vi "click on control.vi"(8 "error in (no error)":errorcluster, 10 "Reference to Button":refnum<vi>, 11 "VI Reference":refnum<vi>) -> (0 "error out":errorcluster)   [LabVIEW 2020, in "ui-testing.lvlib"]
uses:
  ui-testing.lvlib
  User32.dll
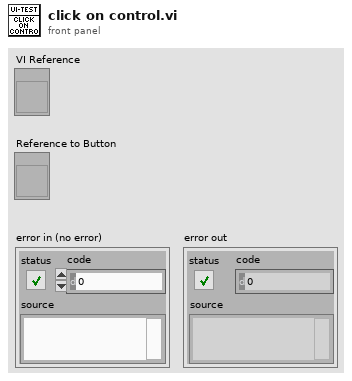
[diagram p1: front panel]
types:
  T1 = typedef "LVRectTypeDef.ctl" = cluster{"left":i16, "top":i16, "right":i16, "bottom":i16}
  T2 = typedef "LVPointTypeDef.ctl" = cluster{"Horizontal":i16, "Vertical":i16}
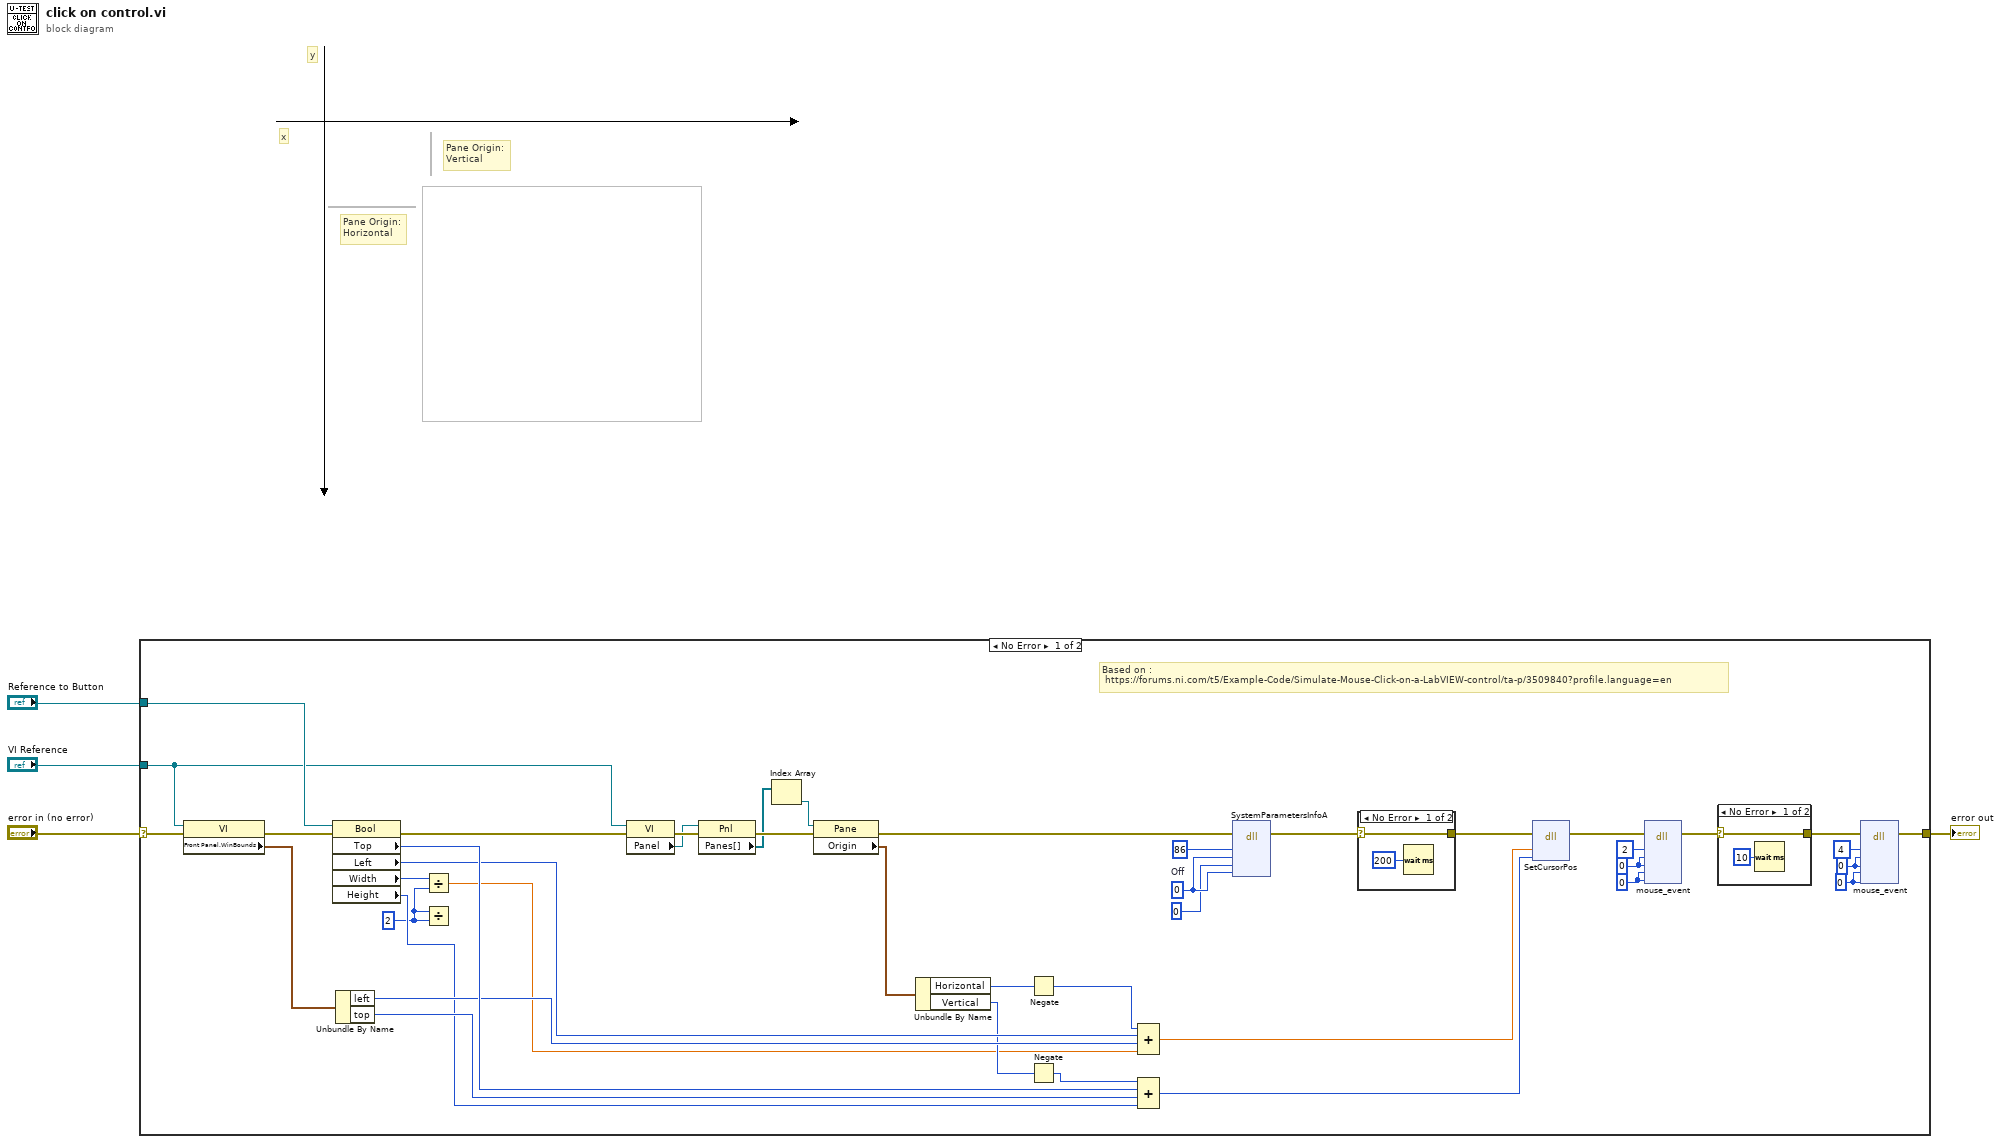
[diagram p0: block diagram]
diagram:
  # "Pane Origin:\nVertical"
  # "Pane Origin:\nHorizontal"
  # "y"
  # "x"
  n1 = case shown="No Error" "error in (no error)" {
    selector: "error in (no error)" -> [w21 w53]
    tunnel: [w32 w53] -> w4
    tunnel: "Reference to Button" -> [w27 _]
    tunnel: "VI Reference" -> [w19 _]
    frame No Error {
      w5 = u32 2 ("y")
      w44 = 0 ("dwExtraInfo")
      w45 = u32 0 ("dwExtraInfo")
      w43 = 0 ("dwExtraInfo")
      w42 = u32 0 ("dwExtraInfo")
      w40 = u32 0  # Off
      # "Based on :\n https://forums.ni.com/t5/Example-Code/Simulate-Mouse-Click-on-a-LabVIEW-control/ta-p/3509840?profile.language=en"
      n2 = property class="VI"(reference=w19, error in=w21) -> (error out=w23:errorcluster, "Front Panel.WinBounds"=w31:T1)  [unwired: 1 out]
      n3 = property on="Property Node" class="Bool"(reference=w27, error in=w23) -> (error out=w22:errorcluster, "Top"=w30:i32, "Left"=w26:i32, "Width"=w8:u32, "Height"=w6:u32)  [unwired: 1 out]
      n4 = Unbundle By Name(w31) -> ("left"=w25:i16, "top"=w29:i16)
      n5 = Divide(x=w8, y=w5) -> (x/y=w7:dbl)
      n6 = Divide(x=w5, y=w5) -> ()  [unwired: 1 out]
      n7 = property class="VI"(reference=w19, error in=w22) -> (error out=w20:errorcluster, "Panel"=w17:refnum<vi>)  [unwired: 1 out]
      n8 = property class="Pnl"(reference=w17, error in=w20) -> (error out=w18:errorcluster, "Panes[]"=w16:refnum<vi>[])  [unwired: 1 out]
      n9 = Index Array(array=w16) -> (element=w14:refnum<vi>)  [unwired: 1 in]
      n10 = property class="Pane"(reference=w14, error in=w18) -> (error out=w15:errorcluster, "Origin"=w13:T2)  [unwired: 1 out]
      n11 = Unbundle By Name(w13) -> ("Horizontal"=w12:i16, "Vertical"=w11:i16)
      n12 = Negate(x=w12) -> (-x=w10:i16)
      n13 = Negate(x=w11) -> (-x=w9:i16)
      n14 = Compound Arithmetic op=ADD(w10, w26, w25, w7) -> (w24:dbl)
      n15 = Compound Arithmetic op=ADD(w9, w30, w29, w6) -> (w28:u32)
      n16 = dll-call lib="User32.dll" fn="SystemParametersInfoA" label="Terminate power-off mode"(error in=w15, "uiAction"=u32 86 ("SPI_GETPOWEROFFACTIVE"), "uiParam"=w40, "pvParam"=0, "fWinIni"=w40) -> (error out=w37:errorcluster)  [unwired: 7 in, 1 out]
      n17 = case shown="No Error" w37 {
        selector: w37 -> [w50 w52]
        tunnel: [w50 w52] -> w36
        frame No Error {
          n18 = Wait (ms)(milliseconds to wait=u32 200) -> ()  [unwired: 1 out]
        }
        frame Error {
        }
      }
      n19 = dll-call lib="User32.dll" fn="SetCursorPos" label="Move mouse"(error in=w36, "dx"=w24, "dy"=w28) -> (error out=w35:errorcluster)  [unwired: 5 in, 1 out]
      n20 = dll-call lib="User32.dll" fn="mouse_event" label="Click"(error in=w35, "dwFlags"=2, "dx"=w43, "dy"=w43, "dwData"=w42, "dwExtraInfo"=w42) -> (error out=w34:errorcluster)  [unwired: 8 in, 1 out]
      n21 = case shown="No Error" w34 {
        selector: w34 -> [w47 w49]
        tunnel: [w47 w49] -> w33
        frame No Error {
          n22 = Wait (ms)(milliseconds to wait=u32 10) -> ()  [unwired: 1 out]
        }
        frame Error {
        }
      }
      n23 = dll-call lib="User32.dll" fn="mouse_event" label="Release"(error in=w33, "dwFlags"=4, "dx"=w44, "dy"=w44, "dwData"=w45, "dwExtraInfo"=w45) -> (error out=w32:errorcluster)  [unwired: 8 in, 1 out]
    }
    frame Error {
    }
  }
  "error out" <- w4
